vi "HMI Main.vi"() -> ()   [LabVIEW 2016]
panel:
  out "size of Final Step array":i32
  out "size of Time array":i32
  out "Time bw two reads":string[](array[string])
  out "Final Step timestamp":timestamp
  out "Final Step timed out?":bool
  out "Time till T_u timestamp":timestamp
  out "Time till T_u timed out?":bool
  out "error out inside loop":errorcluster
  out "error IO":errorcluster
  in  "error in (no error)":errorcluster
  out "Final Step Array":u16[][](array[numeric])
  out "Time till T_u":u32[][](array[numeric])
  in  "stop":bool
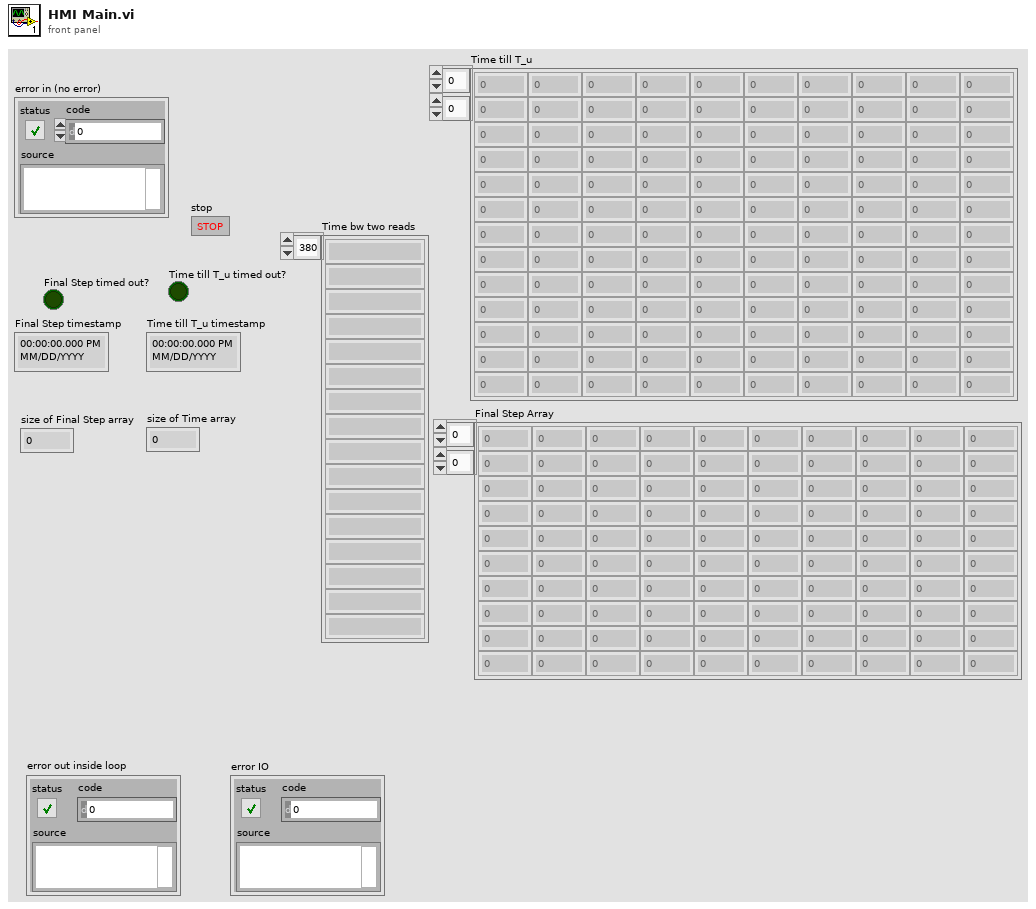
[diagram p1: front panel]
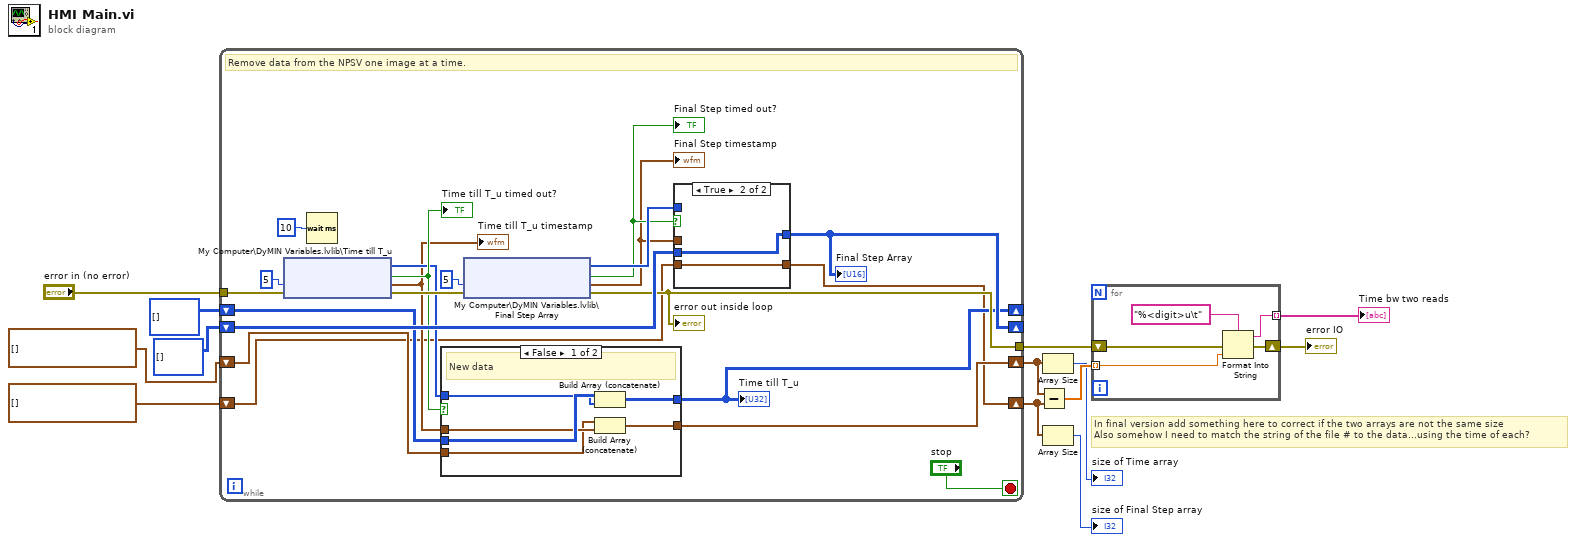
[diagram p0: block diagram]
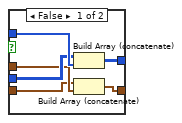
[diagram p2: hidden frame]
diagram:
  # "In final version add something here to correct if the two arrays are not the same size\nAlso somehow I need to match the string of the file # to the data...using the time of each?"
  n1 = while {
    shift-right: [w22] -> _
    shift-left: u32[][] [] -> [w23]
    shift-right: [w31] -> _
    shift-left: u16[][] [] -> [w30]
    tunnel: "error in (no error)" -> [w29]
    tunnel: [w27] -> w7
    shift-right: [w17] -> w4
    shift-left: timestamp[] [] -> [w18]
    shift-right: [w14] -> w1
    shift-left: timestamp[] [] -> [w15]
    stop <- "stop" stop-if-true
    # "Remove data from the NPSV one image at a time."
    n2 = shared-variable "My Computer\\DyMIN Variables.lvlib\\Time till T_u"(error in=w29, 5 ("ms timeout (0)")) -> (w21:u32[], error out=w28:errorcluster, w19:timestamp, w24:bool)
    "Time till T_u timed out?" <- w24
    "Time till T_u timestamp" <- w19
    n3 = Wait (ms)(milliseconds to wait=u32 10) -> ()  [unwired: 1 out]
    n4 = case shown="False" w24 {
      tunnel: w23 -> [w48 w50]
      tunnel: [w46 w50] -> w22
      tunnel: w21 -> [w47 _]
      tunnel: w19 -> [w45 _]
      tunnel: w18 -> [w44 w49]
      tunnel: [w43 w49] -> w17
      frame False {
        # "New data"
        n5 = Build Array (concatenate)(w48, w47) -> (w46:u32[][])
        n6 = Build Array (concatenate)(w44, w45) -> (w43:timestamp[])
      }
      frame True {
        # "No new data"
      }
    }
    "Time till T_u" <- w22
    n7 = shared-variable "My Computer\\DyMIN Variables.lvlib\\Final Step Array"(error in=w28, 5 ("ms timeout (0)")) -> (w32:u16[], error out=w27:errorcluster, w20:bool, w16:timestamp)
    "error out inside loop" <- w27
    "Final Step timed out?" <- w20
    "Final Step timestamp" <- w16
    n8 = case shown="True" w20 {
      tunnel: w32 -> [w40 _]
      tunnel: [w39 w42] -> w31
      tunnel: w30 -> [w38 w42]
      tunnel: w16 -> [w37 _]
      tunnel: w15 -> [w36 w41]
      tunnel: [w35 w41] -> w14
      frame False {
        n9 = Build Array (concatenate)(w38, w40) -> (w39:u16[][])
        n10 = Build Array (concatenate)(w36, w37) -> (w35:timestamp[])
      }
      frame True {
      }
    }
    "Final Step Array" <- w31
  }
  n11 = Subtract(x=w4, y=w1) -> (x-y=w8:dbl[])
  n12 = Array Size(array=w4) -> (size(s)=→"size of Time array":i32)
  n13 = Array Size(array=w1) -> (size(s)=→"size of Final Step array":i32)
  n14 = for {
    tunnel: w8 -> [w55] mode=indexing
    tunnel: [w52] -> w5 mode=indexing
    shift-right: [w51] -> w6
    shift-left: w7 -> [w54]
    n15 = Format Into String(format string="%<digit>u\t", error in=w54, w55) -> (resulting string=w52:string, error out=w51:errorcluster)  [unwired: 1 in]
  }
  "error IO" <- w6
  "Time bw two reads" <- w5
